vi "Write Allow Undefined Names.vi"(8 "error in (no error)":errorcluster, 10 "AllowUndefNames":bool, 11 "DAQChannelName.lvclass in":refnum<class "DAQChannelName.lvclass">) -> (0 "error out":errorcluster, 3 "DAQChannelName.lvclass out":refnum<class "DAQChannelName.lvclass">)   [LabVIEW 2015, in "DAQChannelName.lvclass"]
uses:
  DAQChannelName.lvclass
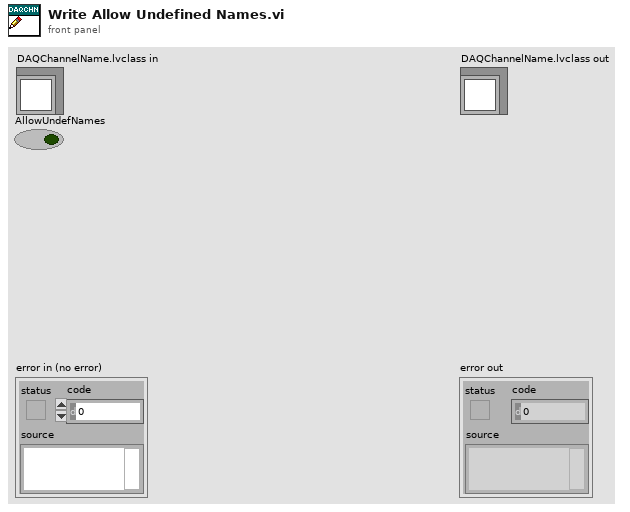
[diagram p1: front panel]
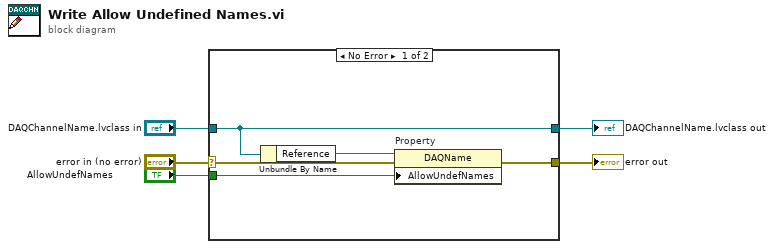
[diagram p0: block diagram]
diagram:
  n1 = case shown="No Error" "error in (no error)" {
    selector: "error in (no error)" -> [w6 w12]
    tunnel: [w10 w12] -> w4
    tunnel: [w8 w11] -> w2
    tunnel: "DAQChannelName.lvclass in" -> [w8 w11]
    tunnel: "AllowUndefNames" -> [w9 _]
    frame No Error {
      n2 = Unbundle By Name(w8) -> ("Reference"=w7:refnum<vi>)
      n3 = property on="Property" class="DAQName"(reference=w7, error in=w6, "AllowUndefNames"=w9) -> (error out=w10:errorcluster)  [unwired: 1 out]
    }
    frame Error {
    }
  }
  "error out" <- w4
  "DAQChannelName.lvclass out" <- w2
